vi "Get_DT_Board_Info_old.vi"() -> (1 "DT Cluster Array":T1[](array[typedef]))   [LabVIEW 2011]
uses:
  Controls/DT_Cluster.ctl
  Controls/DT_Mode.ctl
  Globals/Meas_global.vi
  <userlib>/LV-Link3/PolySubVIs/DtCreateDinChan.vi
  <userlib>/LV-Link3/PolySubVIs/DtOLReadSingle.vi
panel:
  out "Array 6":i32[](array[numeric])
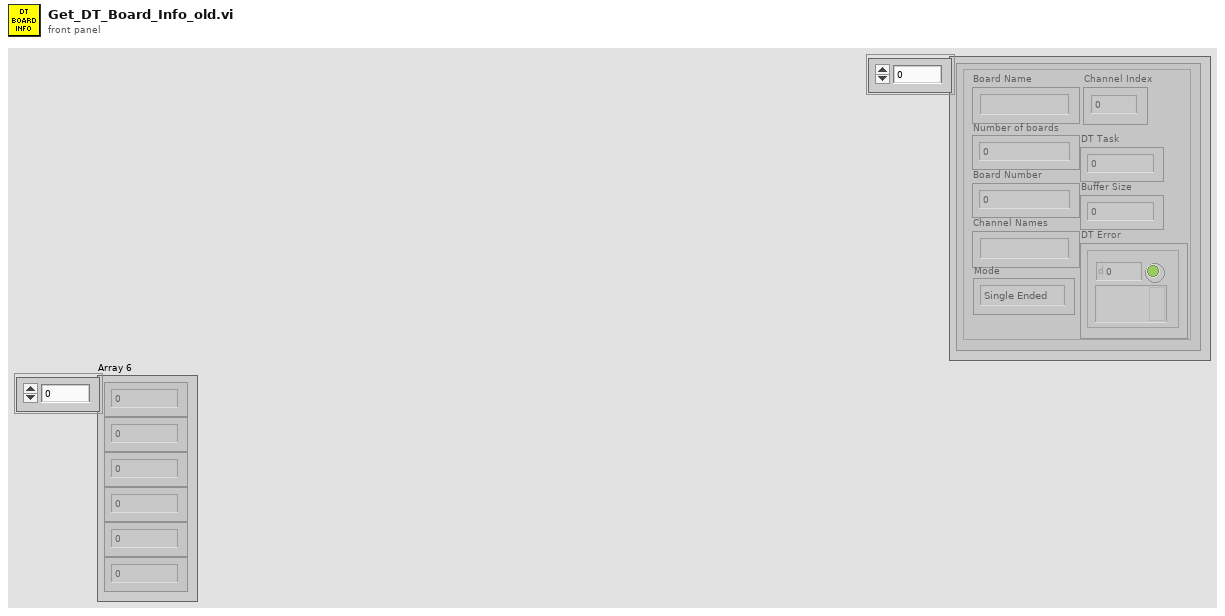
[diagram p1: front panel]
types:
  T1 = typedef "DT_Cluster.ctl" = cluster{"Board Name":string, "Number of boards":u32, "Board Number":u32, "Channel Names":string, "Channel Index":i32[], "DT Task":i32, "DT Error":errorcluster, "Mode":T2, "Buffer Size":u32}
  T2 = typedef "DT_Mode.ctl" = enum16{"Single Ended", "Differential"}
  T3 = typedef "Ch_and_Spans.ctl" = cluster{"high limit (10V)":sgl, "low limit (-10V)":sgl, "Ch No":i16, "Var name":string, "Use Latest Calib":bool}
  T4 = cluster{"Board Number":u32, "Data Translation Board Cluster":T1}
  T5 = cluster{"Board Number":u32, "Data Translation Board Cluster":T1}[]
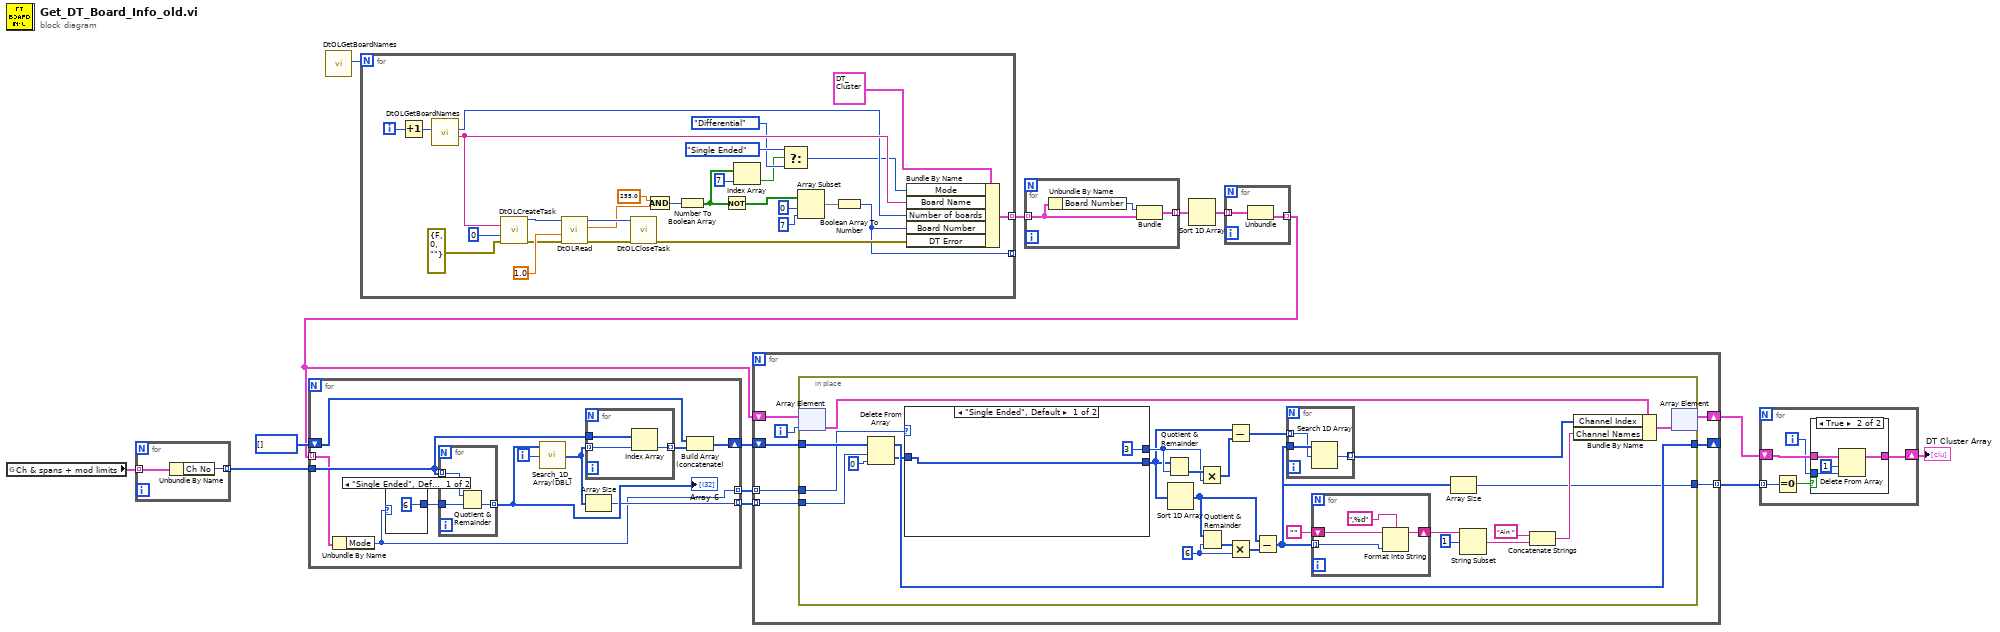
[diagram p0: block diagram]
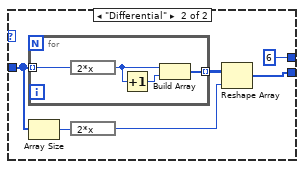
[diagram p3: hidden frame]
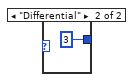
[diagram p4: hidden frame]
diagram:
  n1 = global read "Meas_global.vi" "Ch & spans + mod limits"() -> (w7:T3[])
  n2 = for {
    tunnel: w7 -> [w16] mode=indexing
    tunnel: [w15] -> w6 mode=indexing
    n3 = Unbundle By Name(w16) -> ("Ch No"=w15:i16)
  }
  n4 = call <userlib>:"DtOLGetBoardNames.vi"() -> ("Number of boards"=w14:u32)  [unwired: 9 in, 2 out]
  n5 = for {
    N: w14 -> [_]
    tunnel: [w29] -> w13 mode=indexing
    tunnel: [w17] -> _ mode=indexing
    i -> [w44]
    n6 = Increment(x=w44) -> (x+1=w43:i32)
    n7 = call <userlib>:"DtOLGetBoardNames.vi"("Select Board"=w43) -> ("Board Name"=w33:string, "Number of boards"=w32:u32)  [unwired: 8 in, 1 out]
    n8 = call-poly <userlib>:"DtOLCreateTask.vi"("Board Name"=w33, "Port Number"=u32 0, "error in (no error)"=errorcluster {"status"=FALSE, "code"=0, "source"=""} ("Error Out")) -> ("Task out"=w41:i32, "error out"=w38:errorcluster)  [unwired: 11 in]
    n9 = call-poly <userlib>:"DtOLRead.vi"("error in (no error)"=w38, "Timeout"=1.0 ("Samples Per Channel"), "Task in"=w41) -> ("error out"=w37:errorcluster, "Data Out"=w21:dbl, "Task out"=w36:i32)  [unwired: 6 in]
    n10 = call <userlib>:"DtOLCloseTask.vi"("Error in"=w37, "Task in"=w36) -> ("Error Out"=w19:errorcluster)  [unwired: 9 in]
    n11 = And(x=255.0, y=w21) -> (x .and. y?=w39:i32)
    n12 = Number To Boolean Array(number=w39) -> (Boolean array=w28:bool[])
    n13 = Not(x=w28) -> (.not. x?=w25:bool[])
    n14 = Index Array(array=w28, index=7) -> (element=w26:bool)
    n15 = Select(t=DT_Mode."Single Ended" ("Mode"), s=w26, f=DT_Mode."Differential") -> (s? t:f=w22:T2)
    n16 = Array Subset(array=w25, index=0, length=7) -> (w20:bool[])
    n17 = Boolean Array To Number(Boolean array=w20) -> (number=w17:u32)
    n18 = Bundle By Name(cluster=T1 {"Board Name"="", "Number of boards"=0, "Board Number"=0, "Channel Names"="", "Channel Index"=[], "DT Task"=0, "DT Error"={"status"=FALSE, "code"=0, "source"=""}, "Mode"=enum."Single Ended", "Buffer Size"=0} ("Data Translation Board Cluster"), "Mode"=w22, "Board Name"=w33, "Number of boards"=w32, "Board Number"=w17, "DT Error"=w19) -> (w29:T1)
  }
  n19 = for {
    tunnel: w13 -> [w47] mode=indexing
    tunnel: [w45] -> w12 mode=indexing
    n20 = Unbundle By Name(w47) -> ("Board Number"=w46:u32)
    n21 = Bundle("Board Number"=w46, "Data Translation Board Cluster"=w47) -> (w45:T4)  [unwired: 1 in]
  }
  n22 = Sort 1D Array(array=w12) -> (sorted array=w11:T5)
  n23 = for {
    tunnel: w11 -> [w49] mode=indexing
    tunnel: [w48] -> w4 mode=indexing
    n24 = Unbundle(w49) -> ("Data Translation Board Cluster"=w48:T1)  [unwired: 1 out]
  }
  n25 = for {
    tunnel: w6 -> [w53]
    tunnel: [w57] -> w10 mode=indexing
    shift-right: [w55] -> w8
    shift-left: i32[] [] -> [w54]
    tunnel: w4 -> [w51] mode=indexing
    tunnel: [w50] -> w5 mode=indexing
    i -> [w60]
    n26 = Unbundle By Name(w51) -> ("Mode"=w50:T2)
    n27 = case shown="\"Single Ended\", Default" w50 {
      tunnel: [6 ("y") 3 ("y")] -> w52
      frame "Single Ended", Default {
      }
      frame "Differential" {
      }
    }
    n28 = for {
      tunnel: w53 -> [w67] mode=indexing
      tunnel: [w68] -> w59 mode=indexing
      tunnel: w52 -> [w66]
      n29 = Quotient & Remainder(x=w67, y=w66) -> (floor(x/y)=w68:i32)  [unwired: 1 out]
    }
    "Array 6" <- w59
    n30 = call "Search_1D_Array(DBL).vi"("Array"=w59, "Element Data"=w60) -> ("Indicies of Elements"=w58:i32[])  [unwired: 7 in]
    n31 = for {
      tunnel: w58 -> [w64] mode=indexing
      tunnel: w53 -> [w65]
      tunnel: [w63] -> w56 mode=indexing
      n32 = Index Array(array=w65, index=w64) -> (element=w63:i16)
    }
    n33 = Array Size(array=w58) -> (size(s)=w57:i32)
    n34 = Build Array (concatenate)(w54, w56) -> (w55:i32[])
  }
  n35 = for {
    tunnel: w10 -> [w75] mode=indexing
    shift-right: [w74] -> _
    shift-left: w8 -> [w76]
    shift-right: [w71] -> w2
    shift-left: w4 -> [w72]
    tunnel: w5 -> [w73] mode=indexing
    tunnel: [w69] -> w3 mode=indexing
    i -> [w70]
    n36 = in-place {
      in-place-border: w76 -> [w102]
      in-place-border: w75 -> [w101]
      in-place-border: [w95] -> w74
      in-place-border: w73 -> [w83]
      in-place-border: [w77] -> w69
      w92 = 6 ("offset (0)")
      n37 = in-place-array #1(w72, w70) -> (w82:T1)
      n38 = Delete From Array(array=w102, length=w101, index=0) -> (deleted portion=w93:i32[], array with subset deleted=w95:i32[])
      n39 = case shown="\"Single Ended\", Default" w83 {
        tunnel: w93 -> [w104 w107]
        tunnel: [3 ("offset (0)") 6 ("offset (0)")] -> w86
        tunnel: [w104 w105] -> w84
        frame "Single Ended", Default {
        }
        frame "Differential" {
          n40 = for {
            tunnel: [w113] -> w109 mode=indexing
            tunnel: w107 -> [w111] mode=indexing
            n41 = expression code="2*x"(w111) -> (w112:i32)
            n42 = Increment(x=w112) -> (x+1=w114:i32)
            n43 = Build Array(w112, w114) -> (w113:i32[])
          }
          n44 = Array Size(array=w107) -> (size(s)=w110:i32)
          n45 = expression code="2*x"(w110) -> (w108:i32)
          n46 = Reshape Array(w109, w108) -> (w105:i32[])
        }
      }
      n47 = Quotient & Remainder(x=w84, y=w86) -> (floor(x/y)=w88:i32[])  [unwired: 1 out]
      n48 = Sort 1D Array(array=w84) -> (sorted array=w89:i32[])
      n49 = Multiply(x=w88, y=w86) -> (x*y=w87:i32[])
      n50 = Quotient & Remainder(x=w89, y=w92) -> (floor(x/y)=w90:i32[])  [unwired: 1 out]
      n51 = Subtract(x=w84, y=w87) -> (x-y=w85:i32[])
      n52 = Multiply(x=w90, y=w92) -> (x*y=w91:i32[])
      n53 = Subtract(x=w89, y=w91) -> (x-y=w78:i32[])
      n54 = for {
        tunnel: w78 -> [w121]
        tunnel: w85 -> [w120] mode=indexing
        tunnel: [w119] -> w80 mode=indexing
        n55 = Search 1D Array(1D array=w121, element=w120) -> (index of element=w119:i32)  [unwired: 1 in]
      }
      n56 = for {
        shift-right: [w116] -> w100
        shift-left: "" -> [w117]
        tunnel: w78 -> [w115] mode=indexing
        n57 = Format Into String(format string=",%d", initial string=w117, w115) -> (resulting string=w116:string)  [unwired: 1 in, 1 out]
      }
      n58 = Array Size(array=w78) -> (size(s)=w77:i32)
      n59 = String Subset(string=w100, offset (0)=1) -> (substring=w97:string)  [unwired: 1 in]
      n60 = Concatenate Strings("Ain ", w97) -> (w79:string)
      n61 = Bundle By Name(cluster=w82, "Channel Index"=w80, "Channel Names"=w79) -> (w81:T1)
      n62 = in-place-array #1(w81) -> (w71:T1[])  [unwired: 1 out]
    }
  }
  n63 = for {
    tunnel: w3 -> [w126] mode=indexing
    shift-right: [w123] -> w1
    shift-left: w2 -> [w125]
    i -> [w122]
    n64 = Equal To 0?(x=w126) -> (x = 0?=w124:bool)
    n65 = case shown="True" w124 {
      tunnel: w125 -> [w127 w131]
      tunnel: [w127 w130] -> w123
      tunnel: w122 -> [_ w129]
      frame False {
      }
      frame True {
        n66 = Delete From Array(array=w131, length=1, index=w129) -> (array with subset deleted=w130:T1[])  [unwired: 1 out]
      }
    }
  }
  "DT Cluster Array" <- w1
